vi "Destroy.vi"(8 "error in (no error)":errorcluster, 11 "subscriber in":refnum<class "IcmMessageSubscriber.lvclass">) -> (0 "error out":errorcluster)   [LabVIEW 2017, in "IcmMessageSubscriber.lvclass"]
doc: "Ends the message-bus session for a particular service."
uses:
  <vilib>/addons/InsightCM/MessageBus/MessageSubscriber/IcmMessageSubscriber.lvclass
  <vilib>/addons/InsightCM/MessageBus/MessageSubscriber/IcmMessageSubscriber.lvclass/IcmMessageSubscriber.ctl
  C:/Program Files (x86)/National Instruments/LabVIEW 2017/vi.lib/addons/InsightCM/Binaries/LabviewMessageAdapter.dll
  Binaries/LabviewMessageAdapter.dll
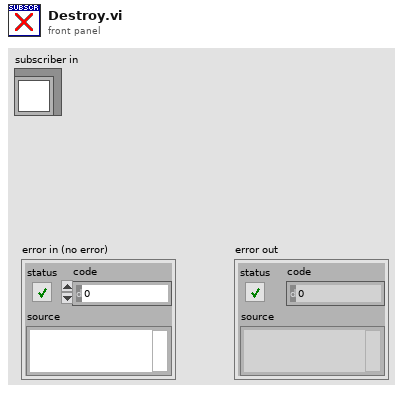
[diagram p1: front panel]
types:
  T1 = typedef "MessageSubscriberDvr.ctl" = refnum<data-value>
  T2 = typedef "MessageSubscriberData.ctl" = cluster{"Subscriber":refnum<k24>}
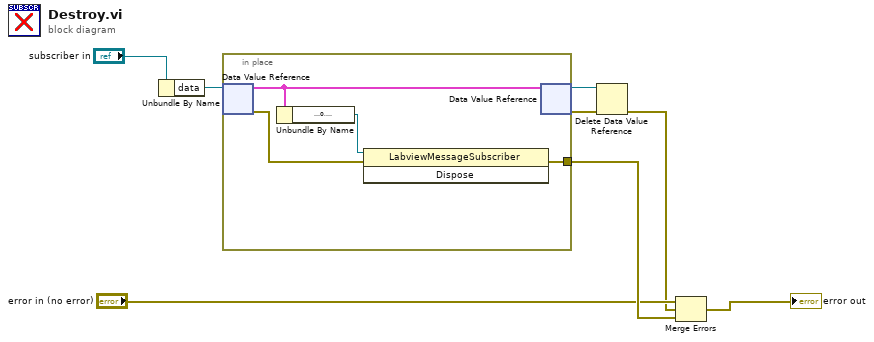
[diagram p0: block diagram]
diagram:
  n1 = Unbundle By Name("subscriber in") -> ("data"=w7:T1)
  n2 = in-place {
    in-place-border: [w9] -> w6
    n3 = in-place-dvr #1(w7) -> (w12:T2, w10:errorcluster)
    n4 = Unbundle By Name(w12) -> ("Subscriber"=w11:refnum<k24>)
    n5 = invoke class="LabviewMessageSubscriber" method="Dispose"(reference=w11, error in=w10) -> (error out=w9:errorcluster)  [unwired: 1 in, 2 out]
    n6 = in-place-dvr #1(w12) -> (w2:T1, w4:errorcluster)
  }
  n7 = Delete Data Value Reference(data value reference=w2, error in=w4) -> (error out=w3:errorcluster)  [unwired: 1 out]
  n8 = Merge Errors("error in (no error)", w3, w6) -> (→"error out":errorcluster)
